vi "End RPC Call.vi"(8 "error in (no error)":errorcluster, 11 "gRPCid":T1) -> (0 "error out":errorcluster)   [LabVIEW 2019, in "Template Server.lvlib" / "Template Server.lvclass"]
uses:
  Template Server.lvclass
  <vilib>/gRPC/LabVIEW gRPC Library/Shared/grpcId.ctl
  <vilib>/gRPC/LabVIEW gRPC Library/gprc-lvsupport-release.lvlib
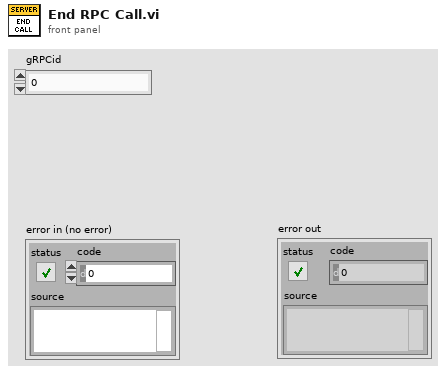
[diagram p1: front panel]
types:
  T1 = typedef "gprc-lvsupport-release.lvlib/grpcId.ctl" = u64
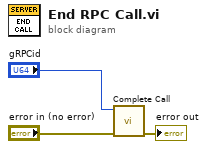
[diagram p0: block diagram]
diagram:
  n1 = call <vilib>:"Complete Call.vi"("gRPCid"="gRPCid", "error in"="error in (no error)") -> ("error out"=→"error out":errorcluster)  [unwired: 8 in]
